vi "DSP Old.vi"(6 "Smooth(F : Don't)":bool, 8 "DSP Parameter":i32[](array[numeric]), 9 "Minus Noise(F : Don't)":bool, 10 "Noise Signal":dbl[](array[numeric]), 11 "Input Signal":dbl[](array[numeric])) -> (3 "DSP signal":dbl[](array[numeric]))   [LabVIEW 2015, in "Digital Signal Processing.lvlib"]
uses:
  Digital Signal Processing.lvlib
  <vilib>/Analysis/3filter.llb/Filter Passband Type.ctl
  <vilib>/Analysis/3filter.llb/Elliptic Filter (DBL).vi
  <vilib>/Analysis/3filter.llb/Butterworth Filter (DBL).vi
  <vilib>/Analysis/NI_AALBase.lvlib
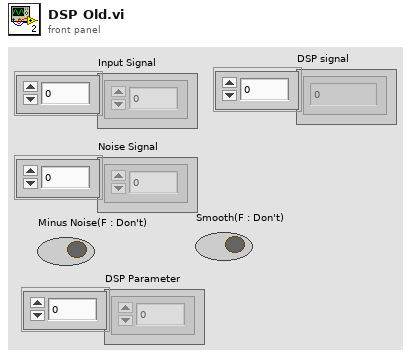
[diagram p1: front panel]
types:
  T1 = typedef "NI_AALBase.lvlib/Filter Passband Type.ctl" = enum32{"Lowpass", "Highpass", "Bandpass", "Bandstop"}
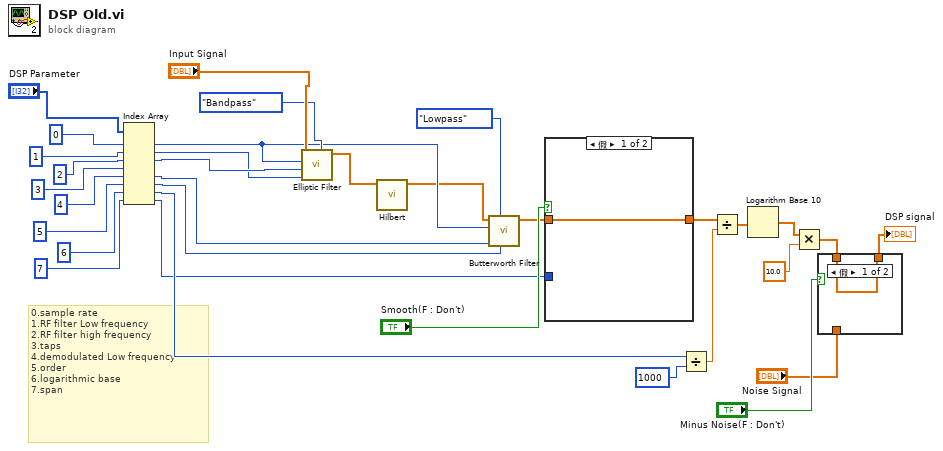
[diagram p0: block diagram]
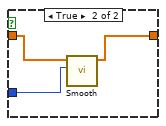
[diagram p2: hidden frame]
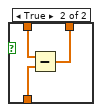
[diagram p3: hidden frame]
diagram:
  # "0.sample rate\n1.RF filter Low frequency\n2.RF filter high frequency\n3.taps\n4.demodulated Low frequency\n5.order\n6.logarithmic base\n7.span"
  n1 = Index Array(array="DSP Parameter", index #1=0 ("索引"), index #2=1 ("索引"), index #3=2 ("索引"), index #4=3 ("索引"), index #5=4 ("索引"), index #6=5 ("索引"), index #7=6 ("索引"), index #8=7 ("索引")) -> (element #1=w15:i32, element #2=w13:i32, element #3=w14:i32, element #5=w23:i32, element #6=w22:i32, element #7=w20:i32, element #8=w6:i32)  [unwired: 1 out]
  n2 = call-poly <vilib>:"Elliptic Filter.vi"("filter type"=Filter_Passband_Type."Bandpass", "low cutoff freq: fl"=w13, "high cutoff freq: fh"=w14, "sampling freq: fs"=w15, "X"="Input Signal") -> ("Filtered X"=w4:dbl[])  [unwired: 5 in, 1 out]
  n3 = call "Hilbert.vi"("X"=w4) -> ("H(X)"=w3:dbl[])  [unwired: 10 in]
  n4 = call-poly <vilib>:"Butterworth Filter.vi"("order"=w22, "filter type"=Filter_Passband_Type."Lowpass", "low cutoff freq: fl"=w23, "sampling freq: fs"=w15, "X"=w3) -> ("Filtered X"=w2:dbl[])  [unwired: 3 in, 1 out]
  n5 = case shown="假" "Smooth(F : Don't)" {
    tunnel: w2 -> [w34 w37]
    tunnel: w6 -> [_ w36]
    tunnel: [w34 w35] -> w5
    frame False {
    }
    frame True {
      n6 = call "Smooth.vi"("SPAN"=w36, "S"=w37) -> ("S_smooth"=w35:dbl[])  [unwired: 9 in]
    }
  }
  n7 = Divide(x=w20, y=1000) -> (x/y=w21:dbl)
  n8 = Divide(x=w5, y=w21) -> (x/y=w18:dbl[])
  n9 = Logarithm Base 10(1:w18) -> (0:w11:dbl[])
  n10 = Multiply(x=w11, y=10.0) -> (x*y=w9:dbl[])
  n11 = case shown="假" "Minus Noise(F : Don't)" {
    tunnel: w9 -> [w38 w41]
    tunnel: "Noise Signal" -> [_ w40]
    tunnel: [w38 w39] -> w1
    frame False {
    }
    frame True {
      n12 = Subtract(x=w41, y=w40) -> (x-y=w39:dbl[])
    }
  }
  "DSP signal" <- w1
